vi "FTW-Actor-OpeningHandshake.vi"(0 "FTW Actor Instance Type":refnum<class "FTW-Actor-Instance.lvclass">, 5 "Initialization Job Sequence":string, 7 "Actor Instance Configuration":string, 11 "error in":errorcluster) -> (4 "FTW Actor Instance":refnum<class "FTW-Actor-Instance.lvclass">, 6 "Incoming Request":refnum<event-registration>, 15 "error out":errorcluster)   [LabVIEW 2015, in "FTW-Actor-Instance.lvclass"]
uses:
  FTW-Actor-Instance.lvclass
  json/core/FTW-JSON-Core-Structure.ctl
  FTW-Actor-Instance.lvclass/FTW-Actor-Instance.ctl
  error/FTW-ERR-ThrowError.vi
  reflection/FTW-Reflection-Type.vi
  time/FTW-Time-RelativeTimer.vi
  error/FTW-ERR-CallChain.vi
  string/FTW-STR-ReplaceWhitespace.vi
  reflection/FTW-Reflection-Array.vi
  error/FTW-ERR-StatusException.vi
  string/FTW-STR-Array-Delimit.vi
  lib/FTW-KernelFilepath.vi
  json/core/FTW-JSON-Core-EncodingFlags.vi
  codegen/xnode/json/fetch/FTW-JSON-Core-GetFlattenedValue.vi
  socket/support/FTW-Socket-Core-LibraryError.vi
  request/FTW-Request-InterpretResponse.vi
  codegen/xnode/FTW-JSON-Fetch.xnode
  codegen/xnode/FTW-Actor-Ask.xnode
  core/type/FTW-Type-Actor-Connector.ctl
panel:
  # "Inputs"
  # "Outputs"
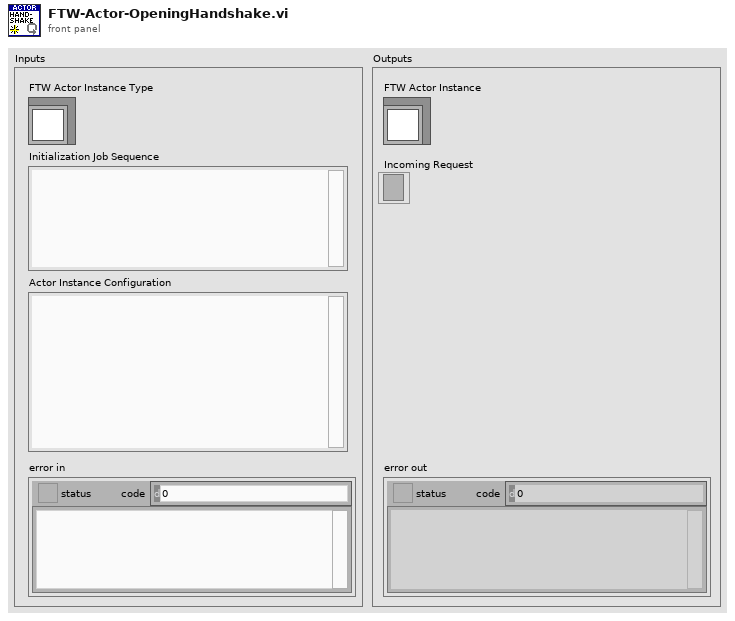
[diagram p1: front panel]
types:
  T1 = cluster{"Identity":string, "InboxAddress":string, "InboxConfiguration":string, "SupervisorAddress":string, "LauncherAddress":string, "DebugEnableInboxLogging":bool, "DebugEnableJobLogging":bool, "LaunchTimeout":i32}
  T2 = typedef "FTW-Type-Actor-Connector.ctl" = refnum<data-value>
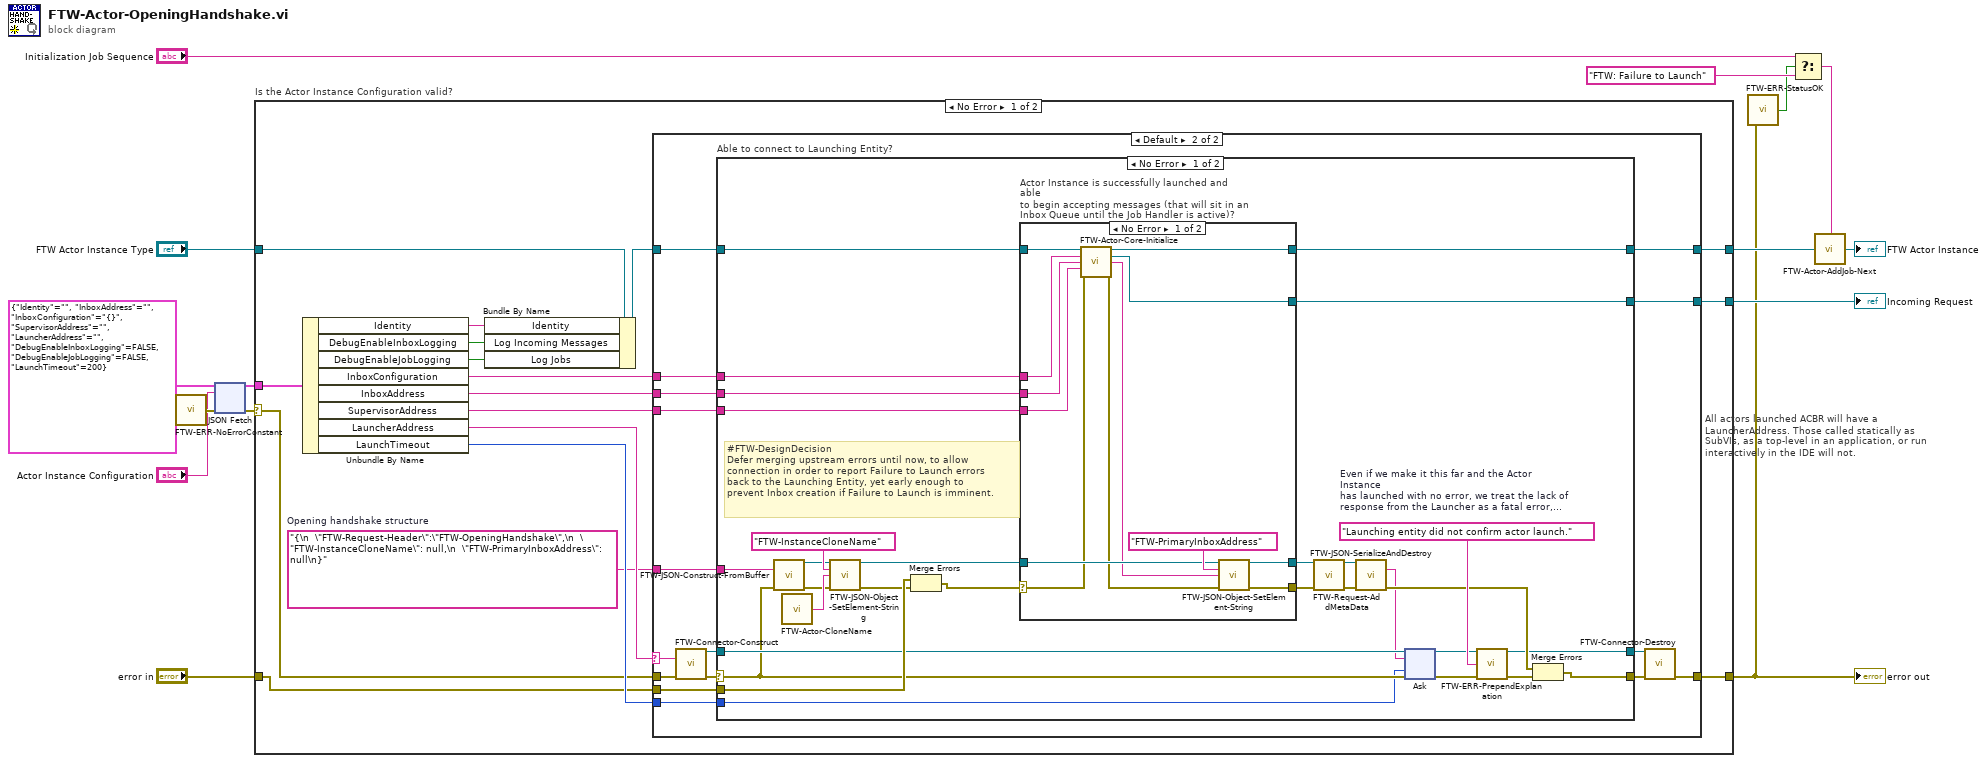
[diagram p0: block diagram]
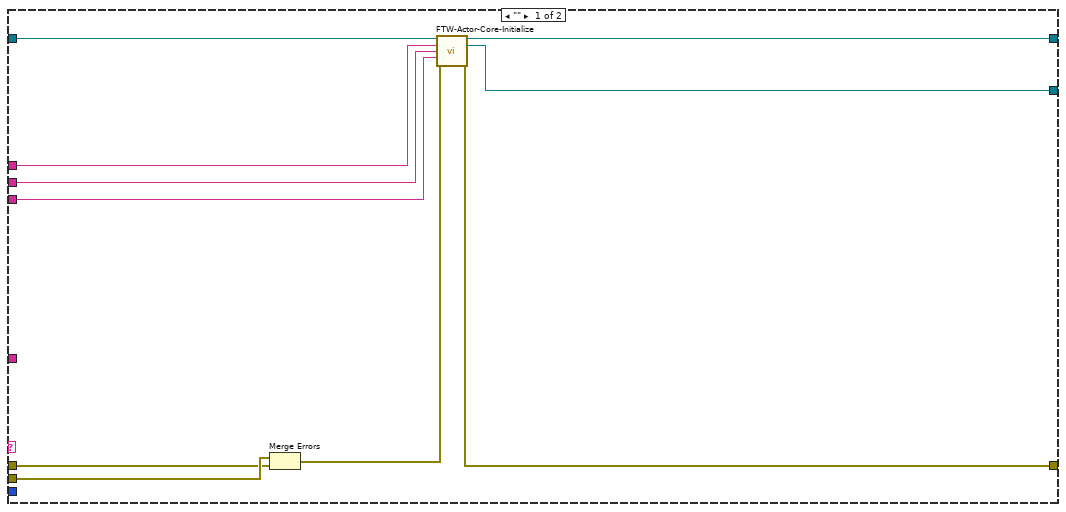
[diagram p2: hidden frame]
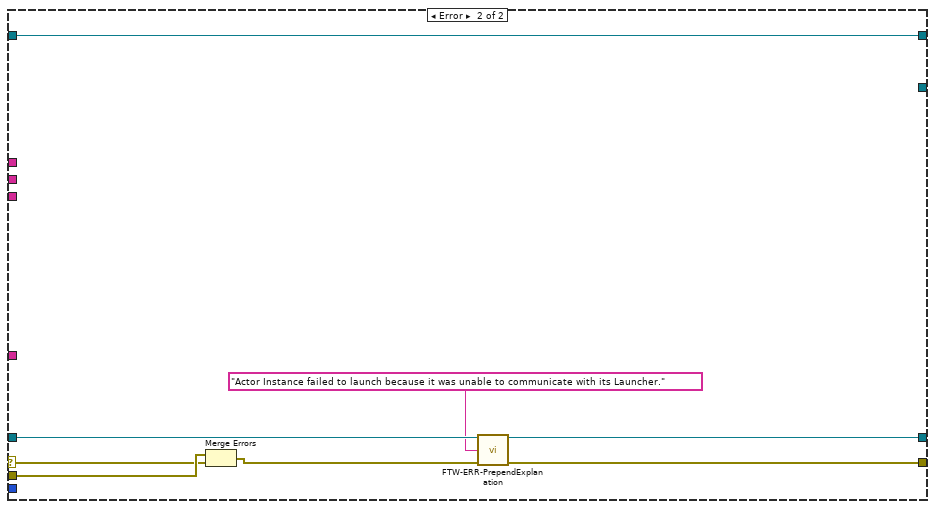
[diagram p4: hidden frame]
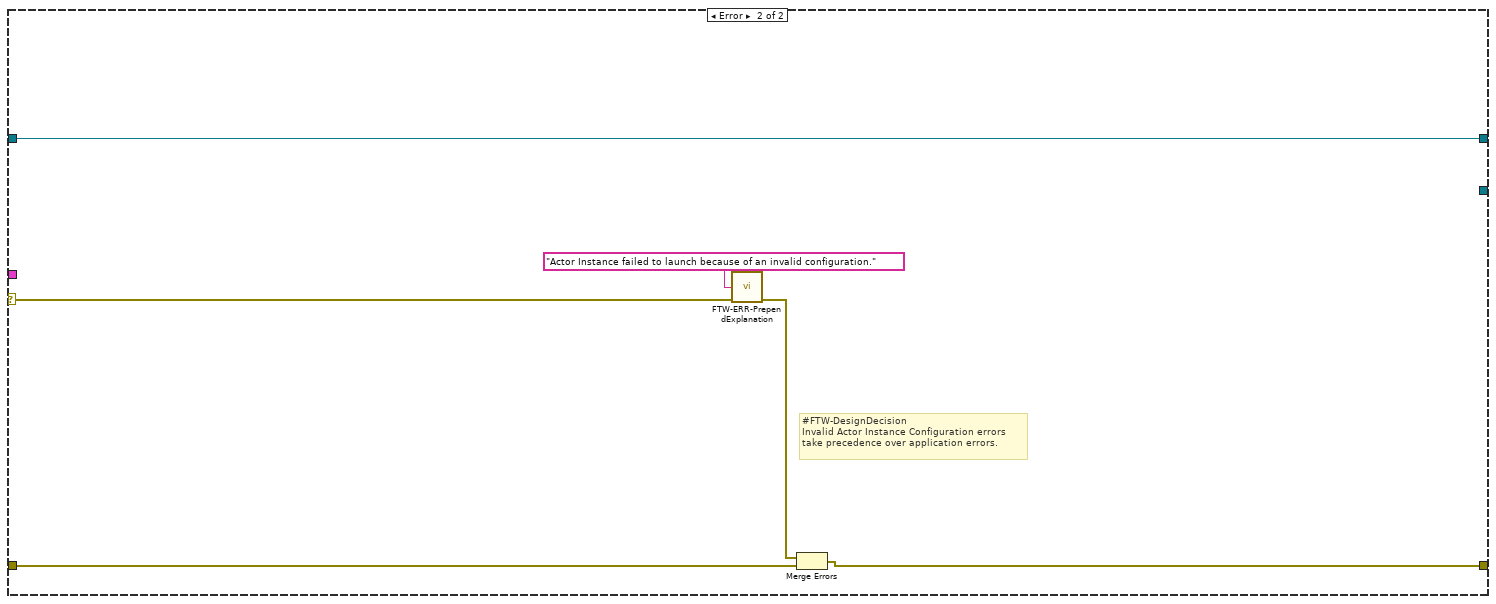
[diagram p5: hidden frame]
diagram:
  n1 = call "FTW-ERR-NoErrorConstant.vi"() -> ("no error"=w3:errorcluster)
  n2 = xnode "JSON Fetch"("Type and Defaults"=T1 {"Identity"="", "InboxAddress"="", "InboxConfiguration"="{}", "SupervisorAddress"="", "LauncherAddress"="", "DebugEnableInboxLogging"=FALSE, "DebugEnableJobLogging"=FALSE, "LaunchTimeout"=200}, "JSON String"="Actor Instance Configuration", "error in"=w3) -> ("Values"=w4:T1, "error out"=w2:errorcluster)  [unwired: 1 in]
  n3 = case "Is the Actor Instance Configuration valid?" shown="No Error" w2 {
    selector: w2 -> [w17 w219]
    tunnel: "FTW Actor Instance Type" -> [w25 w220]
    tunnel: [w27 w215] -> w7
    tunnel: [w32 _] -> w14
    tunnel: [w31 w220] -> w12
    tunnel: w4 -> [w30 _]
    tunnel: "error in" -> [w16 w216]
    frame No Error {
      w19 = "{\n  \"FTW-Request-Header\":\"FTW-OpeningHandshake\",\n  \"FTW-InstanceCloneName\": null,\n  \"FTW-PrimaryInboxAddress\": null\n}"  # Opening handshake structure
      n4 = Unbundle By Name(w30) -> ("Identity"=w23:string, "DebugEnableInboxLogging"=w22:bool, "DebugEnableJobLogging"=w21:bool, "InboxConfiguration"=w20:string, "InboxAddress"=w29:string, "SupervisorAddress"=w18:string, "LauncherAddress"=w26:string, "LaunchTimeout"=w28:i32)
      n5 = Bundle By Name(cluster=w25, "Identity"=w23, "Log Incoming Messages"=w22, "Log Jobs"=w21) -> (w24:refnum<class "FTW-Actor-Instance.lvclass">)
      n6 = case "All actors launched ACBR will have a LauncherAddress. Those called statically as SubVIs, as a top-level in an application, or run interactively in the IDE will not." shown="Default" w26 {
        selector: w26 -> [_ w47]
        tunnel: w24 -> [w42 w58]
        tunnel: [w37 w57] -> w32
        tunnel: [w41 w56] -> w31
        tunnel: w29 -> [w39 w55]
        tunnel: w28 -> [_ w54]
        tunnel: [w38 w49] -> w27
        tunnel: w16 -> [w35 w44]
        tunnel: w19 -> [_ w48]
        tunnel: w20 -> [w40 w46]
        tunnel: w18 -> [w36 w45]
        tunnel: w17 -> [w34 w43]
        frame "" {
          n7 = Merge Errors(w35, w34) -> (w33:errorcluster)
          n8 = call "FTW-Actor-Core-Initialize.vi"("FTW Actor Instance"=w42, "Inbox Configuration"=w40, "Primary Inbox Address"=w39, "Supervisor Address"=w36, "error in"=w33) -> ("FTW Actor Instance out"=w41:refnum<class "FTW-Actor-Instance.lvclass">, "Incoming Request"=w37:refnum<event-registration>, "error out"=w38:errorcluster)  [unwired: 7 in, 1 out]
        }
        frame Default {
          n9 = call "FTW-Connector-Construct.vi"("Remote Inbox Address"=w47, "error in"=w43) -> ("FTW Actor Connector"=w53:T2, "error out"=w52:errorcluster)  [unwired: 12 in]
          n10 = case "Able to connect to Launching Entity?" shown="No Error" w52 {
            selector: w52 -> [w62 w209]
            tunnel: w58 -> [w74 w213]
            tunnel: [w75 w212] -> w50
            tunnel: [w72 _] -> w57
            tunnel: [w71 w213] -> w56
            tunnel: w55 -> [w70 _]
            tunnel: w54 -> [w60 _]
            tunnel: w53 -> [w64 w214]
            tunnel: [w59 w214] -> w51
            tunnel: w48 -> [w78 _]
            tunnel: w46 -> [w73 _]
            tunnel: w45 -> [w69 _]
            tunnel: w44 -> [w68 w210]
            frame No Error {
              w79 = "Launching entity did not confirm actor launch."  # Even if we make it this far and the Actor Instance has launched with no error, we treat the lack of response from the Launcher as a fatal error, such that this Actor Instance does not exist as a renegade.
              # "#FTW-DesignDecision\nDefer merging upstream errors until now, to allow\nconnection in order to report Failure to Launch errors\nback to the Launching Entity, yet early enough to\nprevent Inbox creation if Failure to Launch is imminent."
              n11 = call "FTW-JSON-Construct-FromBuffer.vi"("JSON String (UTF-8)"=w78, "error in"=w62) -> ("JSON Object"=w84:refnum<data-value>, "error out"=w83:errorcluster)  [unwired: 12 in]
              n12 = call "FTW-Actor-CloneName.vi"() -> ("Clone Name"=w87:string)  [unwired: 1 in]
              n13 = call "FTW-JSON-Object-SetElement-String.vi"("JSON Object"=w84, "Key"="FTW-InstanceCloneName", "Value"=w87, "error in"=w83) -> ("JSON Object out"=w82:refnum<data-value>, "error out"=w67:errorcluster)  [unwired: 10 in]
              n14 = Merge Errors(w68, w67) -> (w65:errorcluster)
              n15 = case "Actor Instance is successfully launched and able\nto begin accepting messages (that will sit in an\nInbox Queue until the Job Handler is active)?" shown="No Error" w65 {
                selector: w65 -> [w192 w205]
                tunnel: w82 -> [w203 w206]
                tunnel: [w202 w206] -> w80
                tunnel: w74 -> [w201 w207]
                tunnel: w73 -> [w200 _]
                tunnel: [w199 _] -> w72
                tunnel: [w196 w207] -> w71
                tunnel: w70 -> [w195 _]
                tunnel: w69 -> [w194 _]
                tunnel: [w193 w205] -> w66
                frame No Error {
                  n16 = call "FTW-Actor-Core-Initialize.vi"("FTW Actor Instance"=w201, "Inbox Configuration"=w200, "Primary Inbox Address"=w195, "Supervisor Address"=w194, "error in"=w192) -> ("FTW Actor Instance out"=w196:refnum<class "FTW-Actor-Instance.lvclass">, "Incoming Request"=w199:refnum<event-registration>, "Resolved Primary Inbox Address"=w198:string, "error out"=w197:errorcluster)  [unwired: 7 in]
                  n17 = call "FTW-JSON-Object-SetElement-String.vi"("JSON Object"=w203, "Key"="FTW-PrimaryInboxAddress", "Value"=w198, "error in"=w197) -> ("JSON Object out"=w202:refnum<data-value>, "error out"=w193:errorcluster)  [unwired: 10 in]
                }
                frame Error {
                }
              }
              n18 = call "FTW-Request-AddMetaData.vi"("Response"=w80, "error in"=w66) -> ("Response out"=w86:refnum<data-value>, "error out"=w81:errorcluster)  [unwired: 12 in]
              n19 = call "FTW-JSON-SerializeAndDestroy.vi"("JSON Object"=w86, "error in"=w81) -> ("JSON String (UTF-8)"=w63:string, "error out"=w77:errorcluster)  [unwired: 12 in]
              n20 = xnode "Ask"("FTW Actor Connector"=w64, "Request"=w63, "Timeout"=w60, "error in"=w62) -> ("FTW Actor Connector out"=w59:T2, "error out"=w61:errorcluster)  [unwired: 1 in, 2 out]
              n21 = call "FTW-ERR-PrependExplanation.vi"("Exception Information"=w79, "error in"=w61) -> ("error out"=w76:errorcluster)  [unwired: 13 in]
              n22 = Merge Errors(w77, w76) -> (w75:errorcluster)
            }
            frame Error {
              n23 = Merge Errors(w210, w209) -> (w208:errorcluster)
              n24 = call "FTW-ERR-PrependExplanation.vi"("Exception Information"="Actor Instance failed to launch because it was unable to communicate with its Launcher." ("Error Message"), "error in"=w208) -> ("error out"=w212:errorcluster)  [unwired: 13 in]
            }
          }
          n25 = call "FTW-Connector-Destroy.vi"("FTW Actor Connector"=w51, "error in"=w50) -> ("error out"=w49:errorcluster)  [unwired: 13 in]
        }
      }
    }
    frame Error {
      # "#FTW-DesignDecision\nInvalid Actor Instance Configuration errors\ntake precedence over application errors."
      n26 = call "FTW-ERR-PrependExplanation.vi"("Exception Information"="Actor Instance failed to launch because of an invalid configuration." ("Error Message"), "error in"=w219) -> ("error out"=w218:errorcluster)  [unwired: 13 in]
      n27 = Merge Errors(w218, w216) -> (w215:errorcluster)
    }
  }
  "error out" <- w7
  "Incoming Request" <- w14
  n28 = call "FTW-ERR-StatusOK.vi"("error to check"=w7) -> ("Status OK?"=w8:bool)
  n29 = Select(t="Initialization Job Sequence", s=w8, f="FTW: Failure to Launch") -> (s? t:f=w6:string)
  n30 = call "FTW-Actor-AddJob-Next.vi"("Add Next in Job Queue"=w6, "FTW Actor Instance"=w12) -> ("FTW Actor Instance out"=→"FTW Actor Instance":refnum<class "FTW-Actor-Instance.lvclass">)  [unwired: 2 in]
